vi "SmallAccDAQ.vi"() -> ()   [LabVIEW 2013]
uses:
  <vilib>/Utility/miscctls.llb/LVPointTypeDef.ctl
  <instrlib>/niScope/Controls/niScope vertical coupling.ctl
  <instrlib>/niScope/Controls/niScope trigger coupling.ctl
  <instrlib>/niScope/Controls/niScope trigger slope.ctl
  <instrlib>/niScope/Controls/niScope trigger source.ctl
  Controls/Dust_Event.ctl
  Controls/Signal.ctl
  Controls/Role ID.ctl
  Controls/Hardware ID.ctl
  Controls/Estimate_source.ctl
  Global Variables/Action Items.ctl
  <instrlib>/niScope/Configure/Trigger/niScope Configure Trigger Edge.vi
  <instrlib>/niScope/Acquire/Fetch/niScope Multi Fetch Cluster.vi
panel:
  in  "Clear Errors?":bool
  out "Needle Voltage (kV)":dbl
  out "Number of Events":i32
  in  "Write to Database?":bool
  out "Mass (kg)":dbl
  out "Charge (C)":dbl
  out "Velocity (m/s)":dbl
  out "error out":errorcluster
  in  "stop":bool
  out "Waveform Graph":waveform(dbl)[](graph)
  in  "trigger level":dbl format="%.4f"
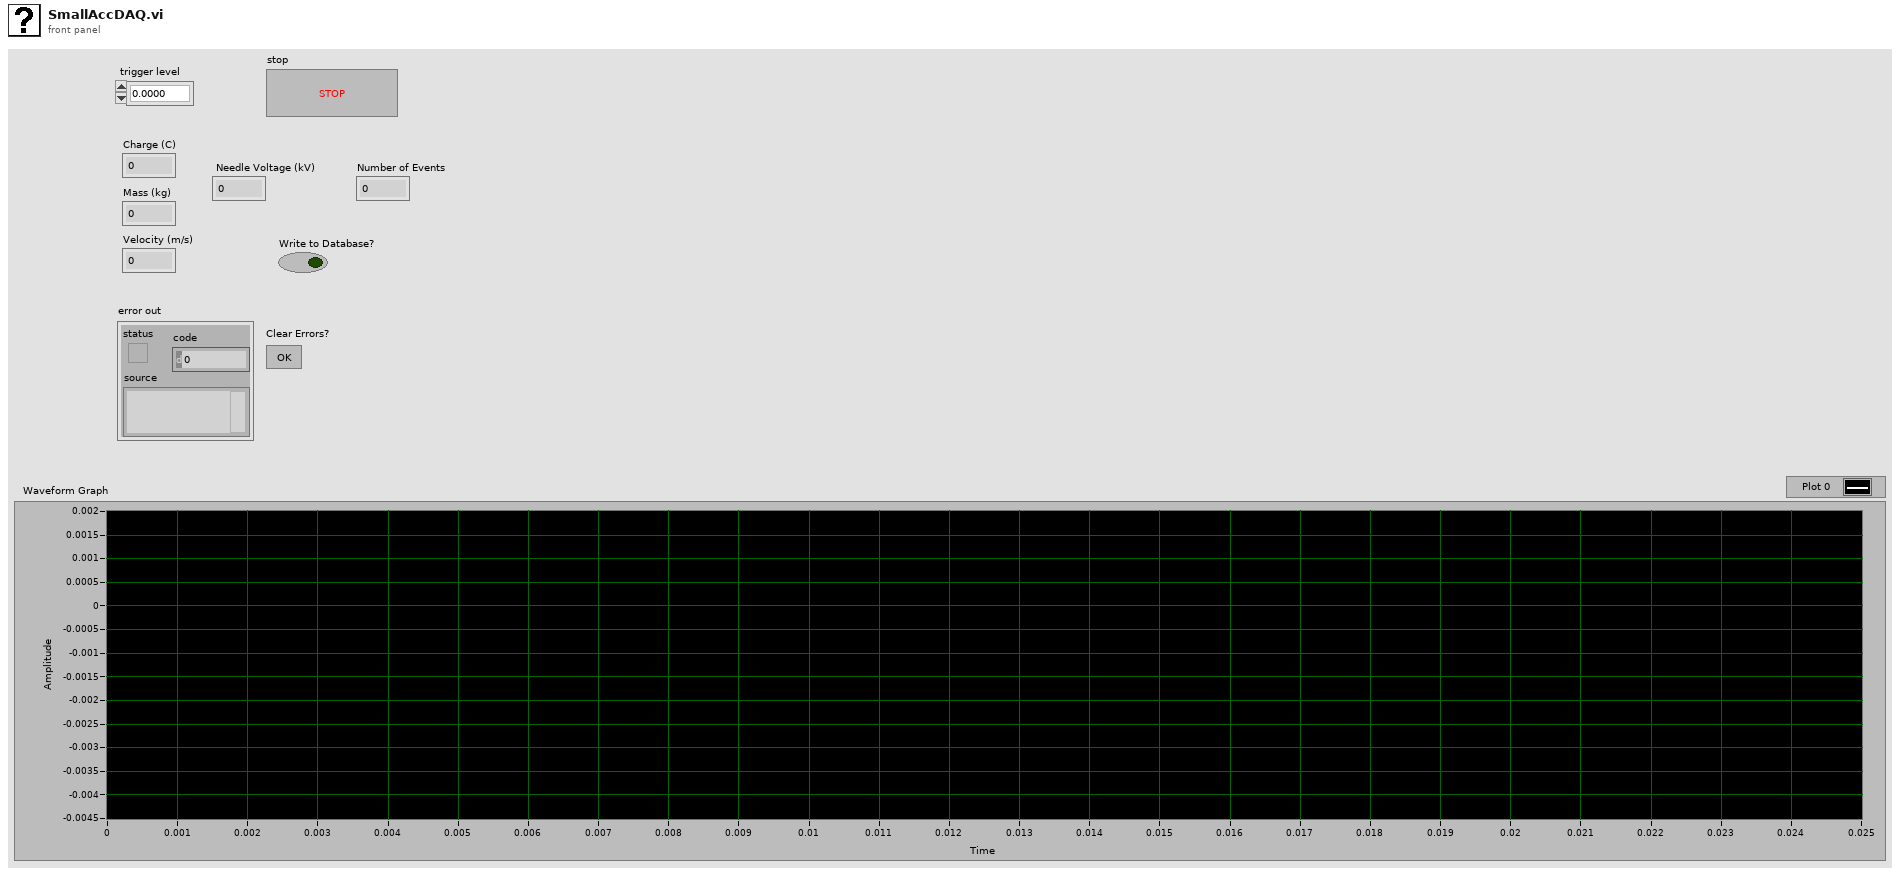
[diagram p1: front panel]
types:
  T1 = typedef "LVPointTypeDef.ctl" = cluster{"Horizontal":i16, "Vertical":i16}
  T2 = typedef "niScope trigger source.ctl" = string
  T3 = cluster{"relativeInitialX":dbl, "xIncrement":dbl, "wfm":dbl[]}[]
  T4 = typedef "Action Items.ctl" = enum16{"Initialize", "Get", "Set"}
  T5 = typedef "Dust_Event.ctl" = cluster{"Time Stamp":timestamp, "Velocity":sgl, "Mass":sgl, "Charge":sgl, "Radius":sgl, "Array":T6[], "Dust Event ID":i64, "Passed_3rd_Detector":bool, "Estimate Source":T9, "Estimate Quality":sgl}
  T6 = typedef "Signal.ctl" = cluster{"Signal ID":i64, "Time Stamp":timestamp, "Dust Event ID":i64, "Role ID":T7, "Data":sgl[], "Signal Length":i32, "dt":sgl, "Offset":dbl, "Hardware ID":T8}
  T7 = typedef "Role ID.ctl" = enum16{"First_Detector", "Second_Detector", "Third_Detector", "LeCroy_CH1", "LeCroy_CH2", "LeCroy_CH3", "LeCroy_CH4", "PSU", "DCS 1", "DCS 2"}
  T8 = typedef "Hardware ID.ctl" = enum16{"Unknown", "CSA 1", "CSA 2", "CSA 3", "CSA 4", "CSA 5", "CSA 6", "DCS 1", "DCS 2"}
  T9 = typedef "Estimate_source.ctl" = i8
  T10 = typedef "niScope trigger slope.ctl" = i32
  T11 = typedef "niScope trigger coupling.ctl" = u16
  T12 = typedef "niScope vertical coupling.ctl" = i32
  T13 = cluster{"relativeInitialX":dbl, "xIncrement":dbl, "wfm":dbl[]}
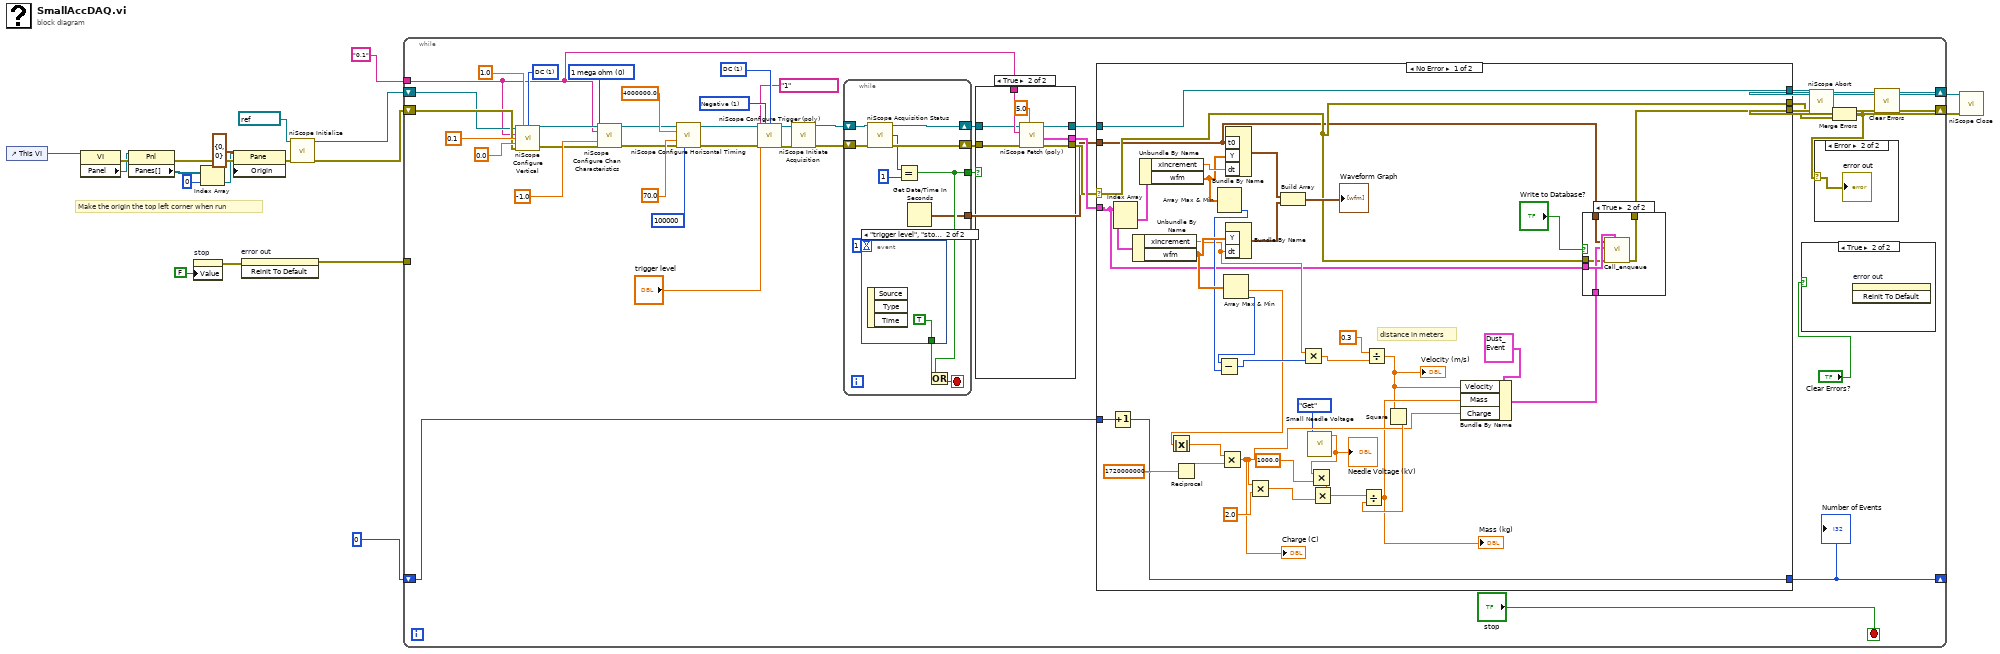
[diagram p0: block diagram]
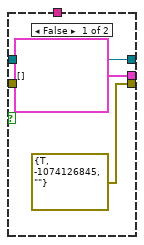
[diagram p2: hidden frame]
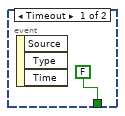
[diagram p3: hidden frame]
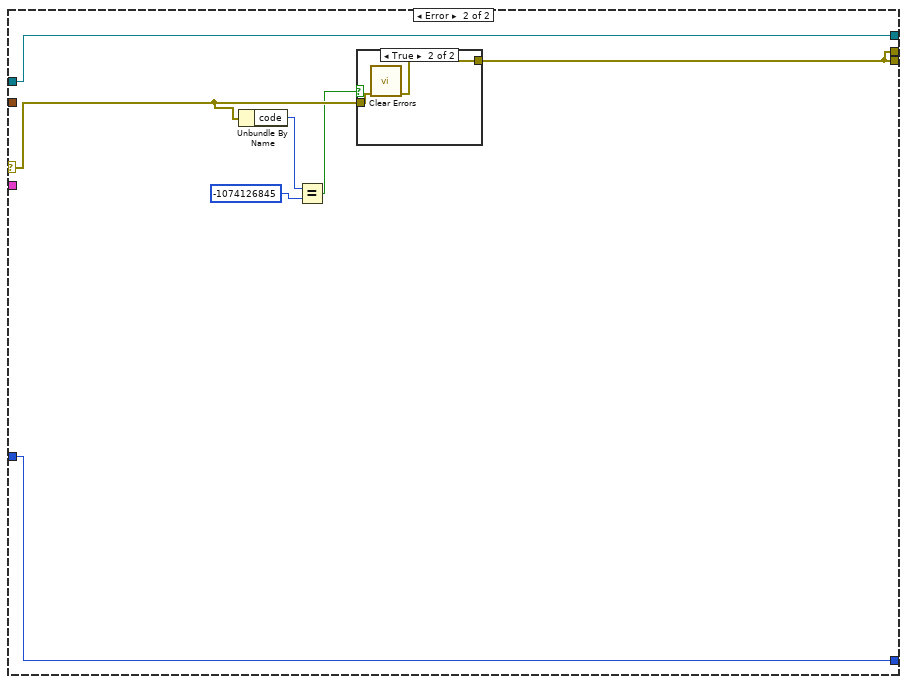
[diagram p7: hidden frame]
diagram:
  # "Make the origin the top left corner when run"
  n1 = control-ref of="This VI"() -> (w10:refnum<vi>)
  n2 = property class="VI"(reference=w10) -> (error out=w17:errorcluster, "Panel"=w11:refnum<vi>)  [unwired: 1 in, 1 out]
  n3 = property class="Pnl"(reference=w11, error in=w17) -> (error out=w16:errorcluster, "Panes[]"=w15:refnum<vi>[])  [unwired: 1 out]
  n4 = property on="stop" class="Bool (strict)"("Value"=FALSE ("stop")) -> (error out=w4:errorcluster)  [unwired: 2 in, 1 out]
  n5 = Index Array(array=w15, index=0) -> (element=w13:refnum<vi>)
  n6 = property class="Pane"(reference=w13, error in=w16, "Origin"=T1 {"Horizontal"=0, "Vertical"=0}) -> (error out=w18:errorcluster)  [unwired: 1 out]
  n7 = invoke on="error out" class="Clust (strict)" method="Reinit To Default"(error in=w4) -> (error out=w5:errorcluster)  [unwired: 2 in, 2 out]
  n8 = call <instrlib>:"niScope Initialize.vi"("resource name"=refnum<k15> "Dev5", "error in"=w18) -> ("instrument handle"=w1:refnum<k15>, "error out"=w2:errorcluster)  [unwired: 12 in]
  n9 = while {
    tunnel: "0,1" ("channels") -> [w40]
    shift-right: [w36] -> w8
    shift-left: w1 -> [w58]
    shift-right: [w28] -> w7
    shift-left: w2 -> [w59]
    shift-right: [w30] -> _
    shift-left: 0 -> [w31]
    tunnel: w5 -> [_]
    stop <- "stop" stop-if-true
    w45 = T10 1 items=["Positive", "Negative"] ("trigger slope")
    w46 = T11 1 items=["AC"=0, "DC"=1, "HF Reject"=3, "LF Reject"=4, "AC Plus HF Reject"=1001] ("trigger coupling")
    w57 = u32 0 items=["1 mega ohm"=0, "50 ohms"=2] ("input impedance")
    w60 = T12 1 items=["AC", "DC", "Ground"] ("vertical coupling")
    n10 = call <instrlib>:"niScope Configure Vertical.vi"("instrument handle"=w58, "probe attenuation"=1.0, "vertical coupling"=w60, "channels"=w40, "vertical range"=0.1, "vertical offset"=0.0, "error in"=w59) -> ("instrument handle out"=w54:refnum<k15>, "error out"=w55:errorcluster)  [unwired: 7 in]
    n11 = call <instrlib>:"niScope Configure Chan Characteristics.vi"("instrument handle"=w54, "channels"=w40, "input impedance"=w57, "maximum input frequency"=-1.0, "error in"=w55) -> ("instrument handle out"=w49:refnum<k15>, "error out"=w50:errorcluster)  [unwired: 9 in]
    n12 = call <instrlib>:"niScope Configure Horizontal Timing.vi"("instrument handle"=w49, "min sample rate"=4000000.0, "reference position"=70.0, "error in"=w50, "min record length"=100000) -> ("instrument handle out"=w48:refnum<k15>, "error out"=w47:errorcluster)  [unwired: 9 in]
    n13 = call-poly <instrlib>:"niScope Configure Trigger (poly).vi"("instrument handle"=w48, "trigger slope"=w45, "trigger coupling"=w46, "trigger source"=T2 "1", "trigger level"="trigger level", "error in"=w47) -> ("instrument handle out"=w42:refnum<k15>, "error out"=w41:errorcluster)  [unwired: 8 in]
    n14 = call <instrlib>:"niScope Initiate Acquisition.vi"("instrument handle"=w42, "error in"=w41) -> ("instrument handle out"=w25:refnum<k15>, "error out"=w24:errorcluster)  [unwired: 12 in]
    n15 = while {
      shift-right: [w81] -> w23
      shift-left: w25 -> [w84]
      shift-right: [w82] -> w22
      shift-left: w24 -> [w83]
      tunnel: [w75] -> w21
      tunnel: [w74] -> w20
      stop <- w76 stop-if-true
      n16 = event shown="[1] \"trigger level\", \"stop\", \"Clear Errors?\": Value Change" {
        selector: _ -> [_ _]
        dyn-events: _ -> [_ _]
        timeout: 1 -> [_ _]
        tunnel: [FALSE TRUE] -> w77
        event Timeout {
          n17 = event-data() -> ()  [unwired: 1 in, 3 out]
        }
        event "trigger level", "stop", "Clear Errors?": Value Change {
          n18 = event-data() -> ()  [unwired: 1 in, 3 out]
        }
      }
      n19 = call <instrlib>:"niScope Acquisition Status.vi"("instrument handle"=w84, "error in"=w83) -> ("instrument handle out"=w81:refnum<k15>, "acquisition status"=w80:i32, "error out"=w82:errorcluster)  [unwired: 11 in]
      n20 = Equal?(x=w80, y=1) -> (x = y?=w75:bool)
      n21 = Get Date/Time In Seconds() -> (seconds since 1Jan1904=w74:timestamp)
      n22 = Or(x=w75, y=w77) -> (x .or. y?=w76:bool)
    }
    n23 = case shown="True" w21 {
      tunnel: w40 -> [_ w73]
      tunnel: [T3 [] ("waveform") w71] -> w39
      tunnel: [w66 w70] -> w38
      tunnel: [errorcluster {"status"=TRUE, "code"=-1074126845, "source"=""} ("error out") w69] -> w32
      tunnel: w23 -> [w66 w68]
      tunnel: w22 -> [_ w67]
      frame False {
      }
      frame True {
        n24 = call-poly <instrlib>:"niScope Fetch (poly).vi"("timeout"=5.0, "error in"=w67, "channels"=w73, "instrument handle"=w68) -> ("error out"=w69:errorcluster, "waveform"=w71:T3, "instrument handle out"=w70:refnum<k15>)  [unwired: 4 in, 1 out]
      }
    }
    n25 = case shown="No Error" w32 {
      selector: w32 -> [w89 w136]
      tunnel: w39 -> [w101 _]
      tunnel: w38 -> [w94 w139]
      tunnel: [w94 w139] -> w37
      tunnel: [w95 w133] -> w33
      tunnel: w31 -> [w93 w134]
      tunnel: [w92 w134] -> w30
      tunnel: [w89 w133] -> w29
      tunnel: w20 -> [w88 _]
      frame No Error {
        # "distance in meters"
        n26 = Increment(x=w93) -> (x+1=w92:i32)
        n27 = Index Array(array=w101) -> (element #1=w126:T13, element #2=w125:T13)  [unwired: 2 in]
        n28 = Unbundle By Name(w125) -> ("xIncrement"=w115:dbl, "wfm"=w120:dbl[])
        n29 = Unbundle By Name(w126) -> ("xIncrement"=w124:dbl, "wfm"=w119:dbl[])
        n30 = Reciprocal(x=17200000000000.0 ("y")) -> (1/x=w109:dbl)
        n31 = Array Max & Min(array=w119) -> (min index (indices)=w117:i32)  [unwired: 3 out]
        n32 = Array Max & Min(array=w120) -> (min value=w112:dbl, min index (indices)=w118:i32)  [unwired: 2 out]
        n33 = Absolute Value(x=w112) -> (abs(x)=w111:dbl)
        n34 = Subtract(x=w118, y=w117) -> (x-y=w116:i32)
        n35 = Multiply(x=w111, y=w109) -> (x*y=w99:dbl)
        "Charge (C)" <- w99
        n36 = Bundle By Name("t0"=w88, "Y"=w119, "dt"=w124) -> (w123:waveform(dbl))  [unwired: 1 in]
        n37 = Bundle By Name("Y"=w120, "dt"=w115) -> (w122:waveform(dbl))  [unwired: 1 in]
        n38 = Multiply(x=w99, y=2.0) -> (x*y=w107:dbl)
        n39 = Build Array(w123, w122) -> (→"Waveform Graph":waveform(dbl)[])
        n40 = Multiply(x=w115, y=w116) -> (x*y=w114:dbl)
        n41 = call "Small Needle Voltage.vi"("Action"=Action_Items."Get") -> ("Output Pelletron Voltage"=w91:dbl)  [unwired: 10 in]
        "Needle Voltage (kV)" <- w91
        n42 = Multiply(x=w91, y=1000.0) -> (x*y=w106:dbl)
        n43 = Multiply(x=w106, y=w107) -> (x*y=w104:dbl)
        n44 = Divide(x=0.3, y=w114) -> (x/y=w97:dbl)
        "Velocity (m/s)" <- w97
        n45 = Square(x=w97) -> (x^2=w103:dbl)
        n46 = Divide(x=w104, y=w103) -> (x/y=w98:dbl)
        "Mass (kg)" <- w98
        n47 = Bundle By Name(cluster=T5 {"Time Stamp"=timestamp(0 s since 1904-01-01), "Velocity"=0.0, "Mass"=0.0, "Charge"=0.0, "Radius"=0.0, "Array"=[], "Dust Event ID"=0, "Passed_3rd_Detector"=FALSE, "Estimate Source"=0, "Estimate Quality"=0.0} ("Input Data"), "Velocity"=w97, "Mass"=w98, "Charge"=w99) -> (w96:T5)
        n48 = case shown="True" "Write to Database?" {
          tunnel: w101 -> [_ w132]
          tunnel: w96 -> [_ w131]
          tunnel: w89 -> [w127 w130]
          tunnel: [w127 w129] -> w95
          tunnel: w88 -> [_ w128]
          frame False {
          }
          frame True {
            n49 = call "Call_enqueue.vi"("Waveform"=w132, "error in"=w130, "Input Data"=w131, "Timestamp"=w128) -> ("error out"=w129:errorcluster)  [unwired: 7 in]
          }
        }
      }
      frame Error {
        n50 = Unbundle By Name(w136) -> ("code"=w138:i32)
        n51 = Equal?(x=w138, y=-1074126845) -> (x = y?=w135:bool)
        n52 = case shown="True" w135 {
          tunnel: [w140 w142] -> w133
          tunnel: w136 -> [w140 w141]
          frame False {
          }
          frame True {
            n53 = call <vilib>:"Clear Errors.vi"("error in (no error)"=w141) -> ("error out"=w142:errorcluster)  [unwired: 6 in]
          }
        }
      }
    }
    "Number of Events" <- w30
    n54 = case shown="True" "Clear Errors?" {
      frame False {
      }
      frame True {
        n55 = invoke on="error out" class="Clust (strict)" method="Reinit To Default"() -> ()  [unwired: 3 in, 3 out]
      }
    }
    n56 = call <instrlib>:"niScope Abort.vi"("instrument handle"=w37, "error in"=w29) -> ("instrument handle out"=w36:refnum<k15>, "error out"=w34:errorcluster)  [unwired: 12 in]
    n57 = Merge Errors(w34, w33) -> (w27:errorcluster)
    n58 = case shown="Error" w27 {
      selector: w27 -> [_ w87]
      frame No Error {
      }
      frame Error {
        "error out" <- w87
      }
    }
    n59 = call <vilib>:"Clear Errors.vi"("error in (no error)"=w27) -> ("error out"=w28:errorcluster)  [unwired: 6 in]
  }
  n60 = call <instrlib>:"niScope Close.vi"("instrument handle"=w8, "error in"=w7) -> ()  [unwired: 13 in, 1 out]
